vi "Create Kernel Module.vi"(7 "Template LVLib Path":path=path "D:/Development/Projects/LQ-CodeGen/templates/LabVIEW/Template.lvlib", 10 "Output Dir":path=path "D:/Development/Projects/LQ-Bindings/src/LabVIEW", 11 "Module Spec. File":path=path "D:/Development/Projects/LQ-CodeGen/data/LQ Core.json") -> (1 "Manifestation Ancestors":T1)   [LabVIEW 2014]
doc: "Copyright (c) 2018 Sze Howe Koh\n\nThis Source Code Form is subject to the terms of the Mozilla Public License, v. 2.0. If a copy of the MPL was not distributed with this file, You can obtain one at http://mozilla.org/MPL/2.0/."
uses:
  Data Structures/Manifestation Ancestors.ctl
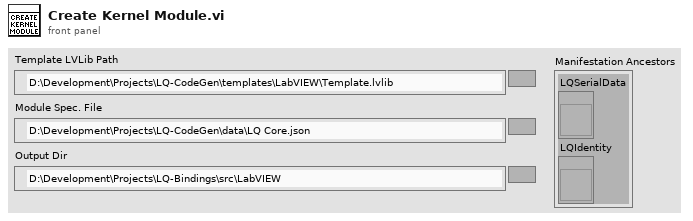
[diagram p1: front panel]
types:
  T1 = typedef "Manifestation Ancestors.ctl" = cluster{"LQSerialData":refnum<vi>, "LQIdentity":refnum<vi>}
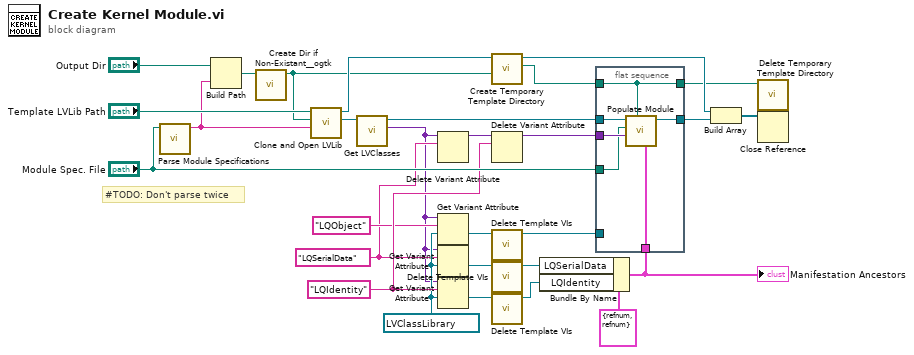
[diagram p0: block diagram]
diagram:
  w6 = refnum<vi> refnum ("Object Ref")
  w4 = "LQSerialData" ("name")
  w8 = "LQIdentity" ("name")
  # "#TODO: Don't parse twice"
  n1 = call "Parse Module Specifications.vi"("Module Spec. File"="Module Spec. File") -> ("Module Name"=w21:string)  [unwired: 6 in, 4 out]
  n2 = Build Path(base path="Output Dir", name or relative path=w21) -> (appended path=w20:path)
  n3 = call <userlib>:"Create Dir if Non-Existant__ogtk.vi"("Directory Path"=w20) -> ("dup Directory Path"=w17:path)  [unwired: 8 in, 2 out]
  n4 = call "Clone and Open LVLib.vi"("Output LVLib Name"=w21, "Output LVLib Dir"=w17, "Template LVLib Path"="Template LVLib Path") -> ("New LVLib"=w29:refnum<vi>, "Template LVLib"=w28:refnum<vi>)  [unwired: 7 in]
  n5 = call "Get LVClasses.vi"("LVLib"=w29) -> ("Class Ref Map"=w3:variant, "LVLib Dup"=w27:refnum<vi>)  [unwired: 9 in]
  n6 = Delete Variant Attribute(6:w4, 7:w3) -> (3:w10:variant)  [unwired: 1 in, 2 out]
  n7 = Get Variant Attribute(Variant=w3, name="LQObject", default value (empty Variant)=w6) -> (value=w5:refnum<vi>)  [unwired: 1 in, 3 out]
  n8 = Get Variant Attribute(Variant=w3, name=w4, default value (empty Variant)=w6) -> (value=w14:refnum<vi>)  [unwired: 1 in, 3 out]
  n9 = Get Variant Attribute(Variant=w3, name=w8, default value (empty Variant)=w6) -> (value=w12:refnum<vi>)  [unwired: 1 in, 3 out]
  n10 = call "Create Temporary Template Directory.vi"("Kernel LVLib Dir"=w17, "Template LVLib"=w28) -> ("Temporary Template Root Dir"=w24:path, "Template LVLib Dup"=w23:refnum<vi>)  [unwired: 8 in]
  n11 = Delete Variant Attribute(6:w8, 7:w10) -> (3:w9:variant)  [unwired: 1 in, 2 out]
  n12 = call "Delete Template VIs.vi"("LVClass"=w5) -> ("LVClass Dup"=w2:refnum<vi>)  [unwired: 10 in]
  n13 = call "Delete Template VIs.vi"("LVClass"=w14) -> ("LVClass Dup"=w13:refnum<vi>)  [unwired: 10 in]
  n14 = call "Delete Template VIs.vi"("LVClass"=w12) -> ("LVClass Dup"=w11:refnum<vi>)  [unwired: 10 in]
  n15 = Bundle By Name(cluster=T1 {"LQSerialData"=refnum, "LQIdentity"=refnum} ("Manifestation Ancestors"), "LQSerialData"=w13, "LQIdentity"=w11) -> (w15:T1)
  "Manifestation Ancestors" <- w15
  n16 = flat-sequence {
    tunnel: w27 -> [w35]
    tunnel: w9 -> [w34]
    tunnel: w24 -> [w31]
    tunnel: "Module Spec. File" -> [w33]
    tunnel: [w32] -> w1
    tunnel: [w31] -> w19
    tunnel: w15 -> [w30]
    tunnel: w2 -> [_]
    frame #0 {
      n17 = call "Populate Module.vi"("Manifestation Ancestors"=w30, "Temporary Template Root Dir"=w31, "Preloaded Module Class Ref Map"=w34, "Module Spec. File"=w33, "Module LVLib"=w35) -> ("Module LVLib Dup"=w32:refnum<vi>)  [unwired: 6 in]
    }
  }
  n18 = Build Array(w23, w1) -> (w26:refnum<vi>[])
  n19 = call "Delete Temporary Template Directory.vi"("Target Template Root Dir"=w19) -> ()  [unwired: 11 in]
  n20 = Close Reference(reference=w26) -> ()  [unwired: 1 in, 1 out]
